vi "find_rects_test.vi"() -> ()   [LabVIEW 2017]
uses:
  gVision/find_rects_parameters.ctl
  gVision/gVision.lvlib
  <vilib>/vision/NI_Vision_Development_Module.lvlib
panel:
  in  "logFileDir":path=path "C:/Users/cfang/Desktop"
  out "Rects":T1(array[cluster])
  in  "find_rects parameters":T2={"nominalWidth"=0.4, "nominalHeight"=0.3, "tolerance"=0.5}
  in  "Field of View":cluster{"fieldOfViewX":sgl, "fieldOfViewY":sgl}={"fieldOfViewX"=1.4, "fieldOfViewY"=1.048}
  out "Number of Rects":i32
  in  "File Path":path=path "C:/Users/cfang/Desktop/nebraska-silicon-lab/pixel-gantry-vision/gVisionLV/Sample Images/TFPX_bond_pad.png"
  out "error out":errorcluster
  out "Image":T3(plugin-control)
  in  "debug":bool
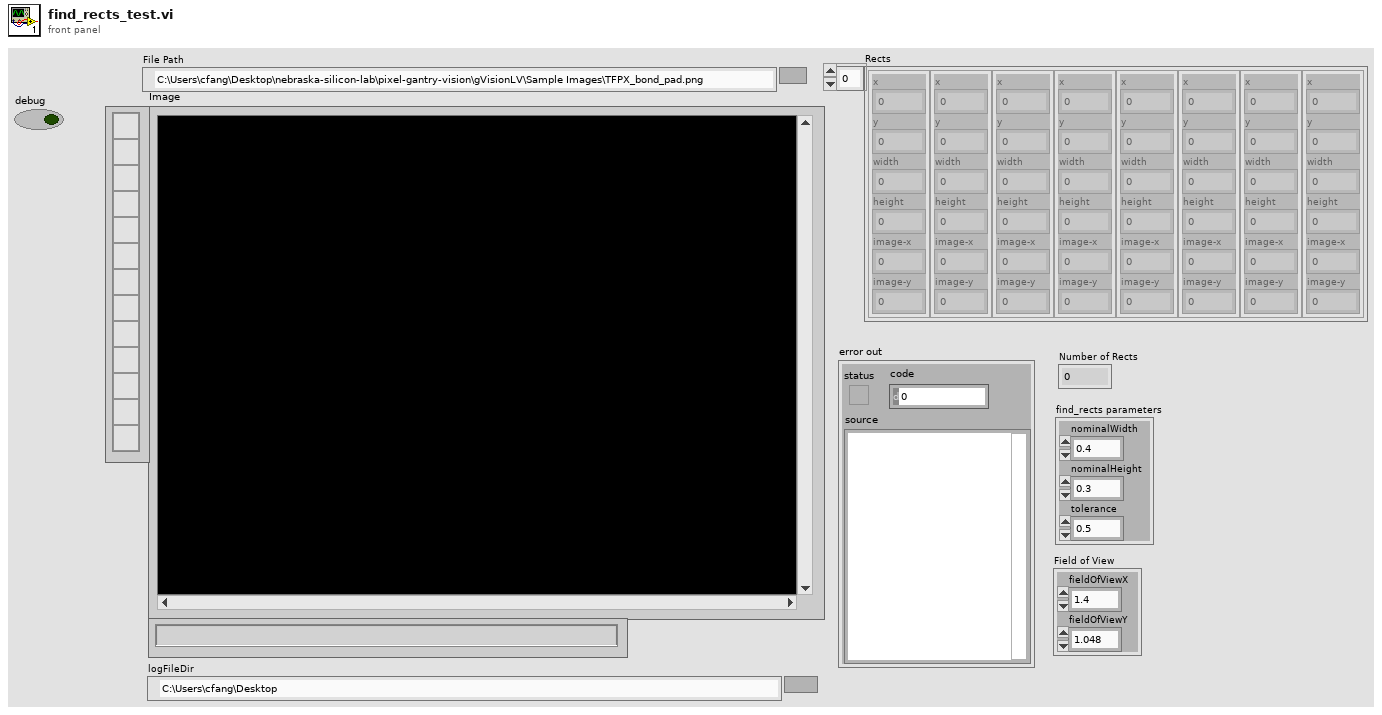
[diagram p1: front panel]
types:
  T1 = cluster{"x":dbl, "y":dbl, "width":dbl, "height":dbl, "image-x":dbl, "image-y":dbl}[]
  T2 = typedef "find_rects_parameters.ctl" = cluster{"nominalWidth":sgl, "nominalHeight":sgl, "tolerance":sgl}
  T3 = typedef "IMAQ Image.ctl" = refnum<image>
  T4 = typedef "Image Type" = u32
  T5 = cluster{"Left":i32, "Top":i32, "Right":i32, "Bottom":i32}
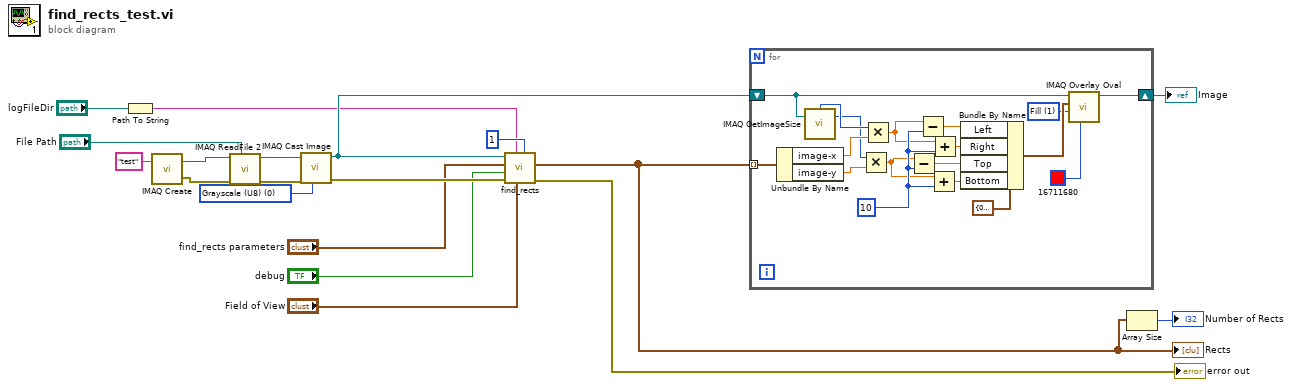
[diagram p0: block diagram]
diagram:
  w13 = T4 0 items=["Grayscale (U8)", "Grayscale (I16)", "Grayscale (SGL)", "Complex (CSG)", "RGB (U32)", "HSL (U32)", "RGB (U64)", "Grayscale (U16)"] ("Image Type")
  n1 = Path To String(path="logFileDir") -> (string=w1:string)
  n2 = call "IMAQ Create"("Image Name"="test") -> ("New Image"=w19:T3, "error out"=w17:errorcluster)  [unwired: 4 in]
  n3 = call "IMAQ ReadFile 2"("File Path"="File Path", "error in (no error)"=w17, "Image"=w19) -> ("error out"=w15:errorcluster, "Image Out"=w14:T3)  [unwired: 4 in, 3 out]
  n4 = call "IMAQ Cast Image"("Image Type"=w13, "error in (no error)"=w15, "Image Src"=w14) -> ("error out"=w10:errorcluster, "Image Dst Out"=w6:T3)  [unwired: 7 in]
  n5 = call "find_rects.vi"("shrinkFactor"=1 ("Shrink Factor"), "Field of View"="Field of View", "logFileDir"=w1, "error in"=w10, "debug"="debug", "find_patches parameters"="find_rects parameters", "Image"=w6) -> ("error out"=→"error out":errorcluster, "Rects"=w3:T1)  [unwired: 3 in]
  "Rects" <- w3
  n6 = for {
    shift-right: [w22] -> w5
    shift-left: w6 -> [w33]
    tunnel: w3 -> [w20] mode=indexing
    w21 = u32 1 items=["Frame", "Fill"] ("Drawing Mode (Frame)")
    w26 = 10
    n7 = Unbundle By Name(w20) -> ("image-x"=w37:dbl, "image-y"=w35:dbl)
    n8 = call "IMAQ GetImageSize"("Image"=w33) -> ("Y Resolution"=w34:i32, "X Resolution"=w36:i32)  [unwired: 3 in, 1 out]
    n9 = Multiply(x=w34, y=w35) -> (x*y=w25:dbl)
    n10 = Multiply(x=w36, y=w37) -> (x*y=w24:dbl)
    n11 = Subtract(x=w25, y=w26) -> (x-y=w27:dbl)
    n12 = Subtract(x=w24, y=w26) -> (x-y=w28:dbl)
    n13 = Add(x=w25, y=w26) -> (x+y=w29:dbl)
    n14 = Add(x=w24, y=w26) -> (x+y=w30:dbl)
    n15 = Bundle By Name(cluster=T5 {"Left"=0, "Top"=0, "Right"=0, "Bottom"=0} ("Bounding Rectangle"), "Left"=w28, "Right"=w30, "Top"=w27, "Bottom"=w29) -> (w23:T5)
    n16 = call "IMAQ Overlay Oval"("Color"=u32 16711680, "Drawing Mode (Frame)"=w21, "Bounding Rectangle"=w23, "Image"=w33) -> ("Image Out"=w22:T3)  [unwired: 6 in, 1 out]
  }
  "Image" <- w5
  n17 = Array Size(array=w3) -> (size(s)=→"Number of Rects":i32)
